vi "VI-File-Explorer.vi"() -> ()   [LabVIEW 2020, in "vi_lib.lvlib"]
uses:
  vi_lib.lvlib
  clLabview/clLabview.lvclass
  clFile/clFile.lvclass
panel:
  in  "new VI-Lib Password":string
  in  "Update LV-Lib Password":bool
  out "File is protected?":bool=TRUE
  out "LV-Lib password (Hex)":string
  out "Icon":picture
  out "busy (*)":bool
  out "Salt (Hex)":string
  out "MD5-Hash 2 (Hex)":string
  out "MD5-Hash 1 (Hex)":string
  out "saving done":bool
  in  "save":bool
  in  "Open":bool
  in  "stop":bool
  out "flags":i32 step=1
  out "stage":u8(ring) items=["development", "alpha", "beta", "release"]
  out "build":u8 step=1
  out "bugfix":u8 step=1
  out "minor":u8 max=99 step=1
  out "major":u8=3 min=1 max=99 step=1
  out "version info":string
  out "version text":string
  in  "save to":path=path "D:/labview/file_in_(free).vi"
  in  "new File Password":string
  in  "open from":path=path "D:/labview/file.vi"
  out "MD5 password (Hex)":string
  # "File password [BDPW]"
  # "VI-File Explorer v.0.11"
  # "by Thomas Zeugner"
  # "Please report bugs and comments to: TomSoftware@gmx.de"
  # "Open"
  # "for LV-Version >= 8"
  # "for LV-Version >= 12"
  # "Save"
  # "File propertys [LVSR]"
  # "File version [vers]"
  # "(*) This is a \"brute force\" version to calc the password Salt, \n      so it might take up to 30sec."
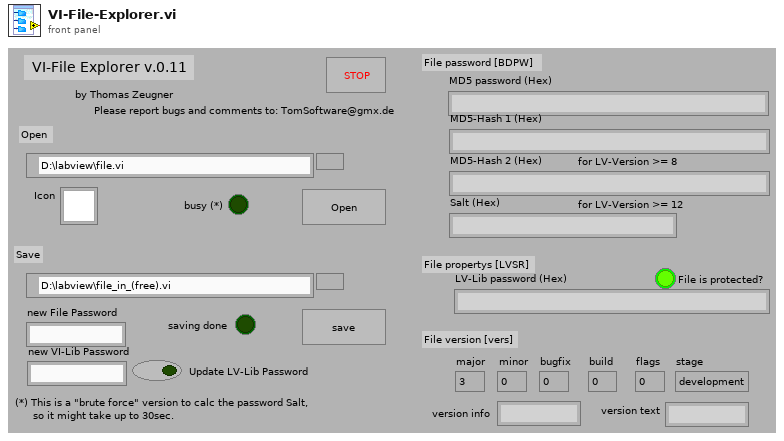
[diagram p1: front panel]
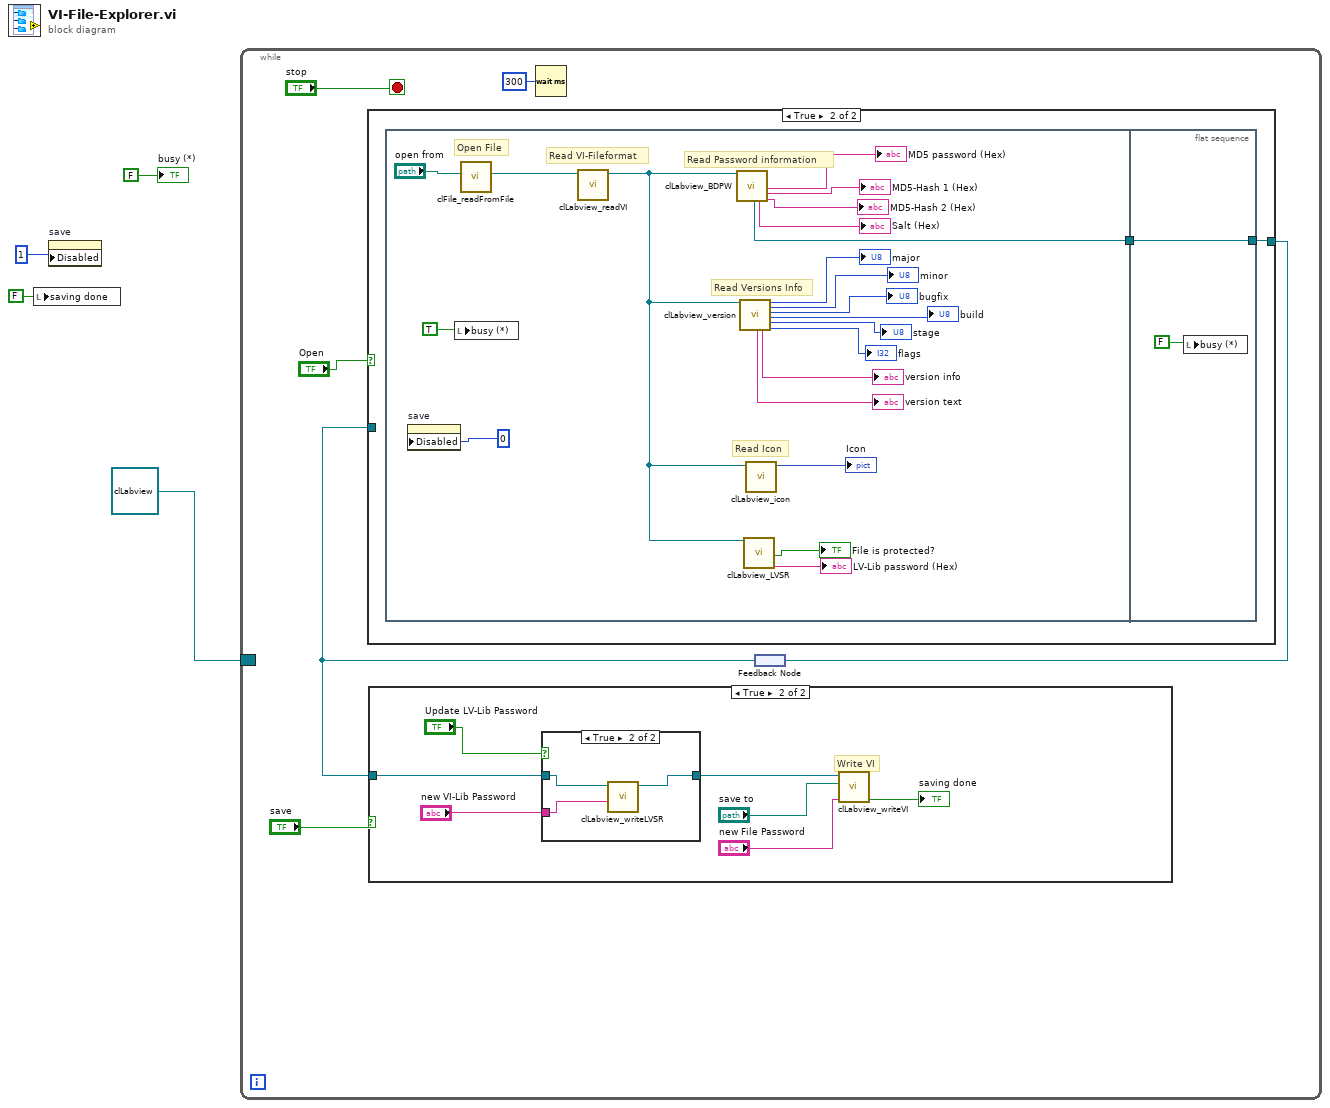
[diagram p0: block diagram]
diagram:
  n1 = local write "saving done"(FALSE ("saving done")) -> ()
  n2 = property on="save" class="Bool"("Disabled"=u8 1) -> ()  [unwired: 2 in, 2 out]
  n3 = while {
    border: refnum<class "clLabview.lvclass"> refnum ("vi_lib.lvlib:clLabview.lvclass 2") -> [_]
    stop <- "stop" stop-if-true
    n4 = Wait (ms)(milliseconds to wait=u32 300) -> ()  [unwired: 1 out]
    n5 = feedback #1() -> (w6:refnum<class "clLabview.lvclass">)
    n6 = case shown="True" "Open" {
      tunnel: [w22 w24] -> w8
      tunnel: w6 -> [w22 _]
      frame False {
      }
      frame True {
        n7 = flat-sequence {
          tunnel: [w30] -> w23
          tunnel: [w47] -> w24
          tunnel: w23 -> [w47]
          frame #0 {
            # "Read Icon"
            # "Read Versions Info"
            # "Read Password information"
            # "Read VI-Fileformat"
            # "Open File"
            n8 = property on="save" class="Bool"("Disabled"=u8 0) -> ()  [unwired: 2 in, 2 out]
            n9 = local write "busy (*)"(TRUE ("busy")) -> ()
            n10 = call "clFile_readFromFile.vi"("file (use dialog)"="open from") -> ("clFileReader.lvclass"=w41:refnum<class "clFileReader.lvclass">)  [unwired: 1 in, 9 out]
            n11 = call "clLabview_readVI.vi"("vi_lib.lvlib:clFileReader.lvclass"=w41) -> ("vi_lib.lvlib:clLabview.lvclass 2"=w27:refnum<class "clLabview.lvclass">)  [unwired: 10 out]
            n12 = call "clLabview_BDPW.vi"("vi_lib.lvlib:clLabview.lvclass"=w27) -> ("vi_lib.lvlib:clLabview.lvclass [Out]"=w30:refnum<class "clLabview.lvclass">, "Salt (Hex)"=→"Salt (Hex)":string, "MD5 password (Hex)"=→"MD5 password (Hex)":string, "MD5-Hash 1  (Hex)"=→"MD5-Hash 1 (Hex)":string, "MD5-Hash 2  (Hex)"=→"MD5-Hash 2 (Hex)":string)  [unwired: 14 out]
            n13 = call "clLabview_version.vi"("vi_lib.lvlib:clLabview.lvclass"=w27) -> ("version_text"=→"version text":string, "version_info"=→"version info":string, "major"=→"major":u8, "minor"=→"minor":u8, "bugfix"=→"bugfix":u8, "build"=→"build":u8, "stage"=→"stage":u8, "flags"=→"flags":i32)  [unwired: 11 out]
            n14 = call "clLabview_LVSR.vi"("vi_lib.lvlib:clLabview.lvclass"=w27) -> ("File is protected?"=→"File is protected?":bool, "MD5 lib Password (Hex)"=→"LV-Lib password (Hex)":string)  [unwired: 17 out]
            n15 = call "clLabview_icon.vi"("vi_lib.lvlib:clLabview.lvclass"=w27) -> ("Icon"=→"Icon":picture)  [unwired: 10 out]
          }
          frame #1 {
            n16 = local write "busy (*)"(FALSE ("busy")) -> ()
          }
        }
      }
    }
    n17 = case shown="True" "save" {
      tunnel: w6 -> [_ w13]
      frame False {
      }
      frame True {
        # "Write VI"
        n18 = case shown="True" "Update LV-Lib Password" {
          tunnel: w13 -> [w18 w21]
          tunnel: [w18 w20] -> w14
          tunnel: "new VI-Lib Password" -> [_ w19]
          frame False {
          }
          frame True {
            n19 = call "clLabview_writeLVSR.vi"("vi_lib.lvlib:clLabview.lvclass"=w21, "new lib Password"=w19) -> ("vi_lib.lvlib:clLabview.lvclass [Out]"=w20:refnum<class "clLabview.lvclass">)  [unwired: 8 out]
          }
        }
        n20 = call "clLabview_writeVI.vi"("vi_lib.lvlib:clLabview.lvclass"=w14, "filename (use dialog)"="save to", "new Password"="new File Password") -> ("no Error"=→"saving done":bool)  [unwired: 7 out]
      }
    }
    n21 = feedback-in #1(w8) -> ()
  }
  "busy (*)" <- FALSE ("busy")
